vi "Read_Parameters.vi"(8 "error in (no error)":errorcluster, 11 "AccelNET.lvlib:TCP.lvclass":refnum<class "TCP.lvclass">) -> (0 "Error Out":errorcluster, 2 "Parameters":T1 {"High\nVoltage (MV)" format="%#.4g"; "Control Reference\nVoltage (MV)" format="%#.4g"; "+ High Voltage\nPS (kV)" format="%#.4g"; "- High Voltage\nPS (kV)" format="%#.4g"; "HV Control\nDifference (kV)" format="%#.4g"; "High Voltage\nPS Setting (kV)" format="%#.4g"; "Chain\nCurrent (uA)" format="%#.4g"; "Column\nCurrent (uA)" format="%#.4g"; "Spark\nLimit" format="%#.0g"; "Spark\nCount" format="%#.0g"; "Lost Charge (uA)" scale=-10.0..10.0; "Spark\nThreshold (MV)" format="%#.4g"; "Radiation (mRad/hr)" step=3.978696e-316 scale=0.02..200.0 scale format="%#.4f"; "Vacuum (Torr)" scale=1e-09..0.001 scale format="%#_6e"})   [LabVIEW 2012, in "AccelNET.lvlib" / "TCP.lvclass"]
uses:
  TCP.lvclass
  Parameters_Indicator.ctl
  Read_Selector.ctl
  Useful_SubVIs.lvlib
  Useful_Controls.lvlib
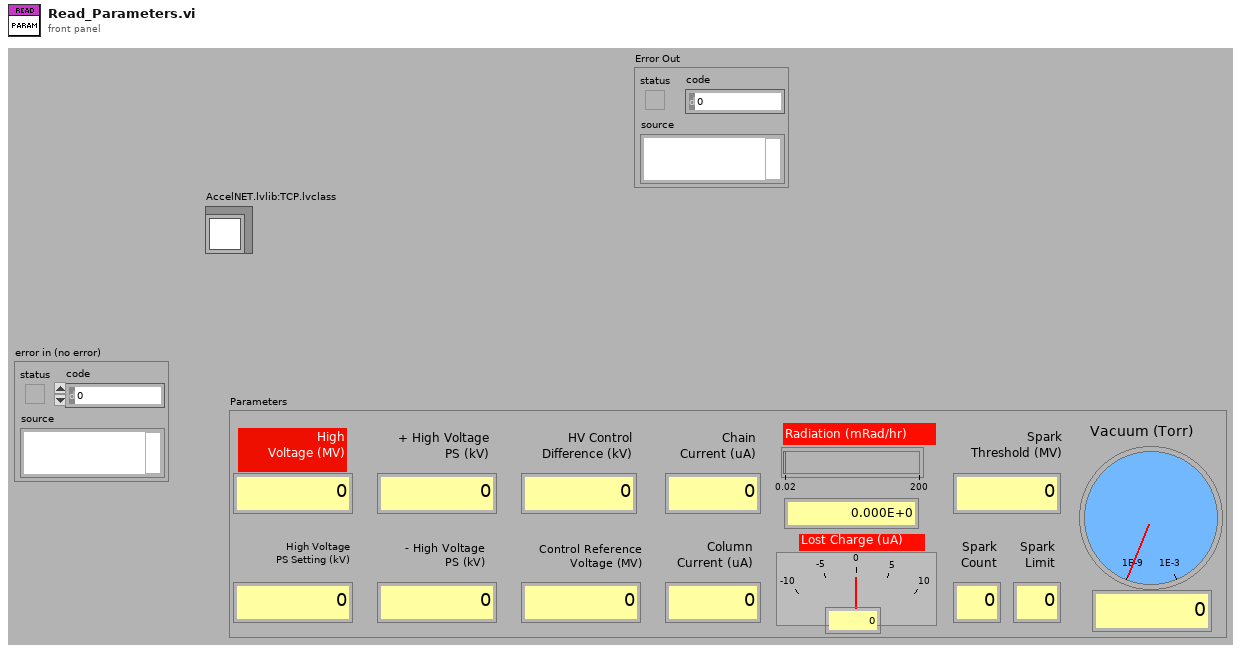
[diagram p1: front panel]
types:
  T1 = typedef "AccelNET.lvlib/Useful_Controls.lvlib/Parameters_Indicator.ctl" = cluster{"Vacuum (Torr)":dbl, "Radiation (mRad/hr)":dbl, "Spark\nThreshold (MV)":dbl, "Lost Charge (uA)":dbl, "Spark\nCount":dbl, "Spark\nLimit":dbl, "Column\nCurrent (uA)":dbl, "Chain\nCurrent (uA)":dbl, "High Voltage\nPS Setting (kV)":dbl, "HV Control\nDifference (kV)":dbl, "- High Voltage\nPS (kV)":dbl, "+ High Voltage\nPS (kV)":dbl, "Control Reference\nVoltage (MV)":dbl, "High\nVoltage (MV)":dbl}
  T2 = typedef "AccelNET.lvlib/Useful_Controls.lvlib/Read_Selector.ctl" = u16
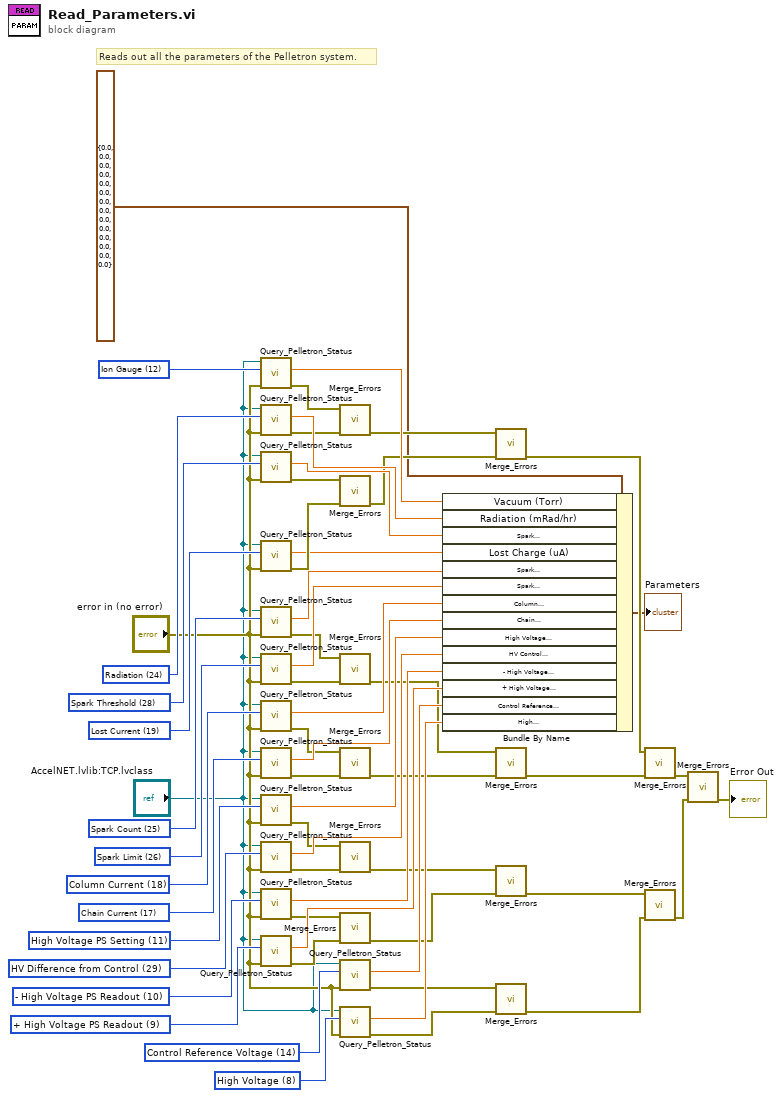
[diagram p0: block diagram]
diagram:
  w46 = T2 8 items=["Facility Key", "Chain Bypass", "Rotating Shaft Bypass", "Facility Interlock", "Pressure Interlock", "Temperature Interlock", "Water Flow Interlock", "Blower Status", "High Voltage", "+ High Voltage PS Readout", "- High Voltage PS Readout", "High Voltage PS Setting", "Ion Gauge", "Ion Filament", "Control Reference Voltage", "Control Mode", "Power Supply", "Chain Current", "Column Current", "Lost Current", "High Voltage Power Supply", "Rotating Shaft", "Chain", "Beamline GV", "Radiation", "Spark Count", "Spark Limit", "Spark Interlock", "Spark Threshold", "HV Difference from Control"] ("Read Selector")
  w47 = T2 14 items=["Facility Key", "Chain Bypass", "Rotating Shaft Bypass", "Facility Interlock", "Pressure Interlock", "Temperature Interlock", "Water Flow Interlock", "Blower Status", "High Voltage", "+ High Voltage PS Readout", "- High Voltage PS Readout", "High Voltage PS Setting", "Ion Gauge", "Ion Filament", "Control Reference Voltage", "Control Mode", "Power Supply", "Chain Current", "Column Current", "Lost Current", "High Voltage Power Supply", "Rotating Shaft", "Chain", "Beamline GV", "Radiation", "Spark Count", "Spark Limit", "Spark Interlock", "Spark Threshold", "HV Difference from Control"] ("Read Selector")
  w48 = T2 9 items=["Facility Key", "Chain Bypass", "Rotating Shaft Bypass", "Facility Interlock", "Pressure Interlock", "Temperature Interlock", "Water Flow Interlock", "Blower Status", "High Voltage", "+ High Voltage PS Readout", "- High Voltage PS Readout", "High Voltage PS Setting", "Ion Gauge", "Ion Filament", "Control Reference Voltage", "Control Mode", "Power Supply", "Chain Current", "Column Current", "Lost Current", "High Voltage Power Supply", "Rotating Shaft", "Chain", "Beamline GV", "Radiation", "Spark Count", "Spark Limit", "Spark Interlock", "Spark Threshold", "HV Difference from Control"] ("Read Selector")
  w49 = T2 10 items=["Facility Key", "Chain Bypass", "Rotating Shaft Bypass", "Facility Interlock", "Pressure Interlock", "Temperature Interlock", "Water Flow Interlock", "Blower Status", "High Voltage", "+ High Voltage PS Readout", "- High Voltage PS Readout", "High Voltage PS Setting", "Ion Gauge", "Ion Filament", "Control Reference Voltage", "Control Mode", "Power Supply", "Chain Current", "Column Current", "Lost Current", "High Voltage Power Supply", "Rotating Shaft", "Chain", "Beamline GV", "Radiation", "Spark Count", "Spark Limit", "Spark Interlock", "Spark Threshold", "HV Difference from Control"] ("Read Selector")
  w50 = T2 29 items=["Facility Key", "Chain Bypass", "Rotating Shaft Bypass", "Facility Interlock", "Pressure Interlock", "Temperature Interlock", "Water Flow Interlock", "Blower Status", "High Voltage", "+ High Voltage PS Readout", "- High Voltage PS Readout", "High Voltage PS Setting", "Ion Gauge", "Ion Filament", "Control Reference Voltage", "Control Mode", "Power Supply", "Chain Current", "Column Current", "Lost Current", "High Voltage Power Supply", "Rotating Shaft", "Chain", "Beamline GV", "Radiation", "Spark Count", "Spark Limit", "Spark Interlock", "Spark Threshold", "HV Difference from Control"] ("Read Selector")
  w51 = T2 11 items=["Facility Key", "Chain Bypass", "Rotating Shaft Bypass", "Facility Interlock", "Pressure Interlock", "Temperature Interlock", "Water Flow Interlock", "Blower Status", "High Voltage", "+ High Voltage PS Readout", "- High Voltage PS Readout", "High Voltage PS Setting", "Ion Gauge", "Ion Filament", "Control Reference Voltage", "Control Mode", "Power Supply", "Chain Current", "Column Current", "Lost Current", "High Voltage Power Supply", "Rotating Shaft", "Chain", "Beamline GV", "Radiation", "Spark Count", "Spark Limit", "Spark Interlock", "Spark Threshold", "HV Difference from Control"] ("Read Selector")
  w52 = T2 17 items=["Facility Key", "Chain Bypass", "Rotating Shaft Bypass", "Facility Interlock", "Pressure Interlock", "Temperature Interlock", "Water Flow Interlock", "Blower Status", "High Voltage", "+ High Voltage PS Readout", "- High Voltage PS Readout", "High Voltage PS Setting", "Ion Gauge", "Ion Filament", "Control Reference Voltage", "Control Mode", "Power Supply", "Chain Current", "Column Current", "Lost Current", "High Voltage Power Supply", "Rotating Shaft", "Chain", "Beamline GV", "Radiation", "Spark Count", "Spark Limit", "Spark Interlock", "Spark Threshold", "HV Difference from Control"] ("Read Selector")
  w53 = T2 18 items=["Facility Key", "Chain Bypass", "Rotating Shaft Bypass", "Facility Interlock", "Pressure Interlock", "Temperature Interlock", "Water Flow Interlock", "Blower Status", "High Voltage", "+ High Voltage PS Readout", "- High Voltage PS Readout", "High Voltage PS Setting", "Ion Gauge", "Ion Filament", "Control Reference Voltage", "Control Mode", "Power Supply", "Chain Current", "Column Current", "Lost Current", "High Voltage Power Supply", "Rotating Shaft", "Chain", "Beamline GV", "Radiation", "Spark Count", "Spark Limit", "Spark Interlock", "Spark Threshold", "HV Difference from Control"] ("Read Selector")
  w54 = T2 26 items=["Facility Key", "Chain Bypass", "Rotating Shaft Bypass", "Facility Interlock", "Pressure Interlock", "Temperature Interlock", "Water Flow Interlock", "Blower Status", "High Voltage", "+ High Voltage PS Readout", "- High Voltage PS Readout", "High Voltage PS Setting", "Ion Gauge", "Ion Filament", "Control Reference Voltage", "Control Mode", "Power Supply", "Chain Current", "Column Current", "Lost Current", "High Voltage Power Supply", "Rotating Shaft", "Chain", "Beamline GV", "Radiation", "Spark Count", "Spark Limit", "Spark Interlock", "Spark Threshold", "HV Difference from Control"] ("Read Selector")
  w55 = T2 25 items=["Facility Key", "Chain Bypass", "Rotating Shaft Bypass", "Facility Interlock", "Pressure Interlock", "Temperature Interlock", "Water Flow Interlock", "Blower Status", "High Voltage", "+ High Voltage PS Readout", "- High Voltage PS Readout", "High Voltage PS Setting", "Ion Gauge", "Ion Filament", "Control Reference Voltage", "Control Mode", "Power Supply", "Chain Current", "Column Current", "Lost Current", "High Voltage Power Supply", "Rotating Shaft", "Chain", "Beamline GV", "Radiation", "Spark Count", "Spark Limit", "Spark Interlock", "Spark Threshold", "HV Difference from Control"] ("Read Selector")
  w56 = T2 19 items=["Facility Key", "Chain Bypass", "Rotating Shaft Bypass", "Facility Interlock", "Pressure Interlock", "Temperature Interlock", "Water Flow Interlock", "Blower Status", "High Voltage", "+ High Voltage PS Readout", "- High Voltage PS Readout", "High Voltage PS Setting", "Ion Gauge", "Ion Filament", "Control Reference Voltage", "Control Mode", "Power Supply", "Chain Current", "Column Current", "Lost Current", "High Voltage Power Supply", "Rotating Shaft", "Chain", "Beamline GV", "Radiation", "Spark Count", "Spark Limit", "Spark Interlock", "Spark Threshold", "HV Difference from Control"] ("Read Selector")
  w57 = T2 28 items=["Facility Key", "Chain Bypass", "Rotating Shaft Bypass", "Facility Interlock", "Pressure Interlock", "Temperature Interlock", "Water Flow Interlock", "Blower Status", "High Voltage", "+ High Voltage PS Readout", "- High Voltage PS Readout", "High Voltage PS Setting", "Ion Gauge", "Ion Filament", "Control Reference Voltage", "Control Mode", "Power Supply", "Chain Current", "Column Current", "Lost Current", "High Voltage Power Supply", "Rotating Shaft", "Chain", "Beamline GV", "Radiation", "Spark Count", "Spark Limit", "Spark Interlock", "Spark Threshold", "HV Difference from Control"] ("Read Selector")
  w58 = T2 24 items=["Facility Key", "Chain Bypass", "Rotating Shaft Bypass", "Facility Interlock", "Pressure Interlock", "Temperature Interlock", "Water Flow Interlock", "Blower Status", "High Voltage", "+ High Voltage PS Readout", "- High Voltage PS Readout", "High Voltage PS Setting", "Ion Gauge", "Ion Filament", "Control Reference Voltage", "Control Mode", "Power Supply", "Chain Current", "Column Current", "Lost Current", "High Voltage Power Supply", "Rotating Shaft", "Chain", "Beamline GV", "Radiation", "Spark Count", "Spark Limit", "Spark Interlock", "Spark Threshold", "HV Difference from Control"] ("Read Selector")
  w59 = T2 12 items=["Facility Key", "Chain Bypass", "Rotating Shaft Bypass", "Facility Interlock", "Pressure Interlock", "Temperature Interlock", "Water Flow Interlock", "Blower Status", "High Voltage", "+ High Voltage PS Readout", "- High Voltage PS Readout", "High Voltage PS Setting", "Ion Gauge", "Ion Filament", "Control Reference Voltage", "Control Mode", "Power Supply", "Chain Current", "Column Current", "Lost Current", "High Voltage Power Supply", "Rotating Shaft", "Chain", "Beamline GV", "Radiation", "Spark Count", "Spark Limit", "Spark Interlock", "Spark Threshold", "HV Difference from Control"] ("Read Selector")
  # "Reads out all the parameters of the Pelletron system."
  n1 = call "Query_Pelletron_Status.vi"("error in (no error)"="error in (no error)", "Read Selector"=w59, "AccelNET.lvlib:TCP.lvclass"="AccelNET.lvlib:TCP.lvclass") -> ("error out"=w18:errorcluster, "Data Out"=w44:dbl)  [unwired: 7 in]
  n2 = call "Query_Pelletron_Status.vi"("error in (no error)"="error in (no error)", "Read Selector"=w58, "AccelNET.lvlib:TCP.lvclass"="AccelNET.lvlib:TCP.lvclass") -> ("error out"=w19:errorcluster, "Data Out"=w43:dbl)  [unwired: 7 in]
  n3 = call "Query_Pelletron_Status.vi"("error in (no error)"="error in (no error)", "Read Selector"=w57, "AccelNET.lvlib:TCP.lvclass"="AccelNET.lvlib:TCP.lvclass") -> ("error out"=w20:errorcluster, "Data Out"=w42:dbl)  [unwired: 7 in]
  n4 = call "Query_Pelletron_Status.vi"("error in (no error)"="error in (no error)", "Read Selector"=w56, "AccelNET.lvlib:TCP.lvclass"="AccelNET.lvlib:TCP.lvclass") -> ("error out"=w21:errorcluster, "Data Out"=w1:dbl)  [unwired: 7 in]
  n5 = call "Query_Pelletron_Status.vi"("error in (no error)"="error in (no error)", "Read Selector"=w55, "AccelNET.lvlib:TCP.lvclass"="AccelNET.lvlib:TCP.lvclass") -> ("error out"=w22:errorcluster, "Data Out"=w41:dbl)  [unwired: 7 in]
  n6 = call "Query_Pelletron_Status.vi"("error in (no error)"="error in (no error)", "Read Selector"=w54, "AccelNET.lvlib:TCP.lvclass"="AccelNET.lvlib:TCP.lvclass") -> ("error out"=w23:errorcluster, "Data Out"=w40:dbl)  [unwired: 7 in]
  n7 = call "Query_Pelletron_Status.vi"("error in (no error)"="error in (no error)", "Read Selector"=w53, "AccelNET.lvlib:TCP.lvclass"="AccelNET.lvlib:TCP.lvclass") -> ("error out"=w24:errorcluster, "Data Out"=w39:dbl)  [unwired: 7 in]
  n8 = call "Query_Pelletron_Status.vi"("error in (no error)"="error in (no error)", "Read Selector"=w52, "AccelNET.lvlib:TCP.lvclass"="AccelNET.lvlib:TCP.lvclass") -> ("error out"=w25:errorcluster, "Data Out"=w38:dbl)  [unwired: 7 in]
  n9 = call "Query_Pelletron_Status.vi"("error in (no error)"="error in (no error)", "Read Selector"=w51, "AccelNET.lvlib:TCP.lvclass"="AccelNET.lvlib:TCP.lvclass") -> ("error out"=w26:errorcluster, "Data Out"=w37:dbl)  [unwired: 7 in]
  n10 = call "Query_Pelletron_Status.vi"("error in (no error)"="error in (no error)", "Read Selector"=w50, "AccelNET.lvlib:TCP.lvclass"="AccelNET.lvlib:TCP.lvclass") -> ("error out"=w27:errorcluster, "Data Out"=w36:dbl)  [unwired: 7 in]
  n11 = call "Query_Pelletron_Status.vi"("error in (no error)"="error in (no error)", "Read Selector"=w49, "AccelNET.lvlib:TCP.lvclass"="AccelNET.lvlib:TCP.lvclass") -> ("error out"=w28:errorcluster, "Data Out"=w35:dbl)  [unwired: 7 in]
  n12 = call "Query_Pelletron_Status.vi"("error in (no error)"="error in (no error)", "Read Selector"=w48, "AccelNET.lvlib:TCP.lvclass"="AccelNET.lvlib:TCP.lvclass") -> ("error out"=w29:errorcluster, "Data Out"=w34:dbl)  [unwired: 7 in]
  n13 = call "Merge_Errors.vi"("Error 2"=w19, "Error 1"=w18) -> ("Error Out"=w17:errorcluster)  [unwired: 9 in]
  n14 = call "Merge_Errors.vi"("Error 2"=w21, "Error 1"=w20) -> ("Error Out"=w16:errorcluster)  [unwired: 9 in]
  n15 = call "Merge_Errors.vi"("Error 2"=w23, "Error 1"=w22) -> ("Error Out"=w15:errorcluster)  [unwired: 9 in]
  n16 = call "Merge_Errors.vi"("Error 2"=w25, "Error 1"=w24) -> ("Error Out"=w14:errorcluster)  [unwired: 9 in]
  n17 = call "Merge_Errors.vi"("Error 2"=w27, "Error 1"=w26) -> ("Error Out"=w13:errorcluster)  [unwired: 9 in]
  n18 = call "Merge_Errors.vi"("Error 2"=w29, "Error 1"=w28) -> ("Error Out"=w12:errorcluster)  [unwired: 9 in]
  n19 = call "Query_Pelletron_Status.vi"("error in (no error)"="error in (no error)", "Read Selector"=w47, "AccelNET.lvlib:TCP.lvclass"="AccelNET.lvlib:TCP.lvclass") -> ("error out"=w30:errorcluster, "Data Out"=w33:dbl)  [unwired: 7 in]
  n20 = call "Query_Pelletron_Status.vi"("error in (no error)"="error in (no error)", "Read Selector"=w46, "AccelNET.lvlib:TCP.lvclass"="AccelNET.lvlib:TCP.lvclass") -> ("error out"=w31:errorcluster, "Data Out"=w32:dbl)  [unwired: 7 in]
  n21 = Bundle By Name(cluster=T1 {"Vacuum (Torr)"=0.0, "Radiation (mRad/hr)"=0.0, "Spark\nThreshold (MV)"=0.0, "Lost Charge (uA)"=0.0, "Spark\nCount"=0.0, "Spark\nLimit"=0.0, "Column\nCurrent (uA)"=0.0, "Chain\nCurrent (uA)"=0.0, "High Voltage\nPS Setting (kV)"=0.0, "HV Control\nDifference (kV)"=0.0, "- High Voltage\nPS (kV)"=0.0, "+ High Voltage\nPS (kV)"=0.0, "Control Reference\nVoltage (MV)"=0.0, "High\nVoltage (MV)"=0.0} ("Parameters"), "Vacuum (Torr)"=w44, "Radiation (mRad/hr)"=w43, "Spark\nThreshold (MV)"=w42, "Lost Charge (uA)"=w1, "Spark\nCount"=w41, "Spark\nLimit"=w40, "Column\nCurrent (uA)"=w39, "Chain\nCurrent (uA)"=w38, "High Voltage\nPS Setting (kV)"=w37, "HV Control\nDifference (kV)"=w36, "- High Voltage\nPS (kV)"=w35, "+ High Voltage\nPS (kV)"=w34, "Control Reference\nVoltage (MV)"=w33, "High\nVoltage (MV)"=w32) -> (→"Parameters":T1)
  n22 = call "Merge_Errors.vi"("Error 2"=w16, "Error 1"=w17) -> ("Error Out"=w9:errorcluster)  [unwired: 9 in]
  n23 = call "Merge_Errors.vi"("Error 2"=w14, "Error 1"=w15) -> ("Error Out"=w8:errorcluster)  [unwired: 9 in]
  n24 = call "Merge_Errors.vi"("Error 2"=w12, "Error 1"=w13) -> ("Error Out"=w10:errorcluster)  [unwired: 9 in]
  n25 = call "Merge_Errors.vi"("Error 2"=w31, "Error 1"=w30) -> ("Error Out"=w11:errorcluster)  [unwired: 9 in]
  n26 = call "Merge_Errors.vi"("Error 2"=w8, "Error 1"=w9) -> ("Error Out"=w7:errorcluster)  [unwired: 9 in]
  n27 = call "Merge_Errors.vi"("Error 2"=w11, "Error 1"=w10) -> ("Error Out"=w6:errorcluster)  [unwired: 9 in]
  n28 = call "Merge_Errors.vi"("Error 2"=w6, "Error 1"=w7) -> ("Error Out"=→"Error Out":errorcluster)  [unwired: 9 in]
